vi "Prompt Unflatten Test Parameters.vi"(9 "error in (no error)":errorcluster, 10 "Parameter String":string) -> (1 "error out":errorcluster, 2 "Prompt Test Parameters":T2, 5 "Test Version":string)   [LabVIEW 2011]
uses:
  TypeDefs/Prompt Test Parameters.ctl
  Test Return Parameter.ctl
  TypeDefs/Prompt Test Parameters v1.0-1.4.ctl
  TypeDefs/Prompt Test Parameters v1.5-1.6.ctl
  TypeDefs/Prompt Test Parameters v1.7.ctl
  TypeDefs/Prompt Test Parameters v1.8.ctl
panel:
  in  "Return Parameter":T1
  out "Parameter Variant":variant
  in  "Required Instruments":string[](array[string])
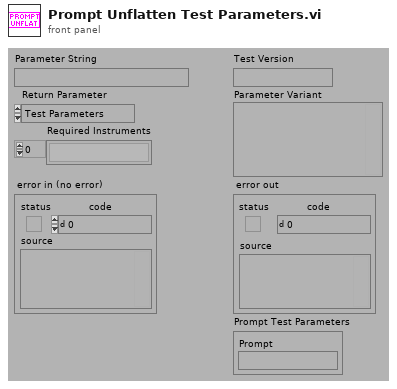
[diagram p1: front panel]
types:
  T1 = typedef "Test Return Parameter.ctl" = enum16{"Test Parameters", "Required Instruments", "Datasheets", "QuickMode"}
  T2 = typedef "Prompt Test Parameters.ctl" = cluster{"Prompt":string}
  T3 = typedef "Prompt Test Parameters v1.0-1.4.ctl" = cluster{"Prompt":string, "Tag":string}
  T4 = typedef "Prompt Test Parameters v1.5-1.6.ctl" = cluster{"Tag":string, "Prompt":string, "Reports":cluster{"Reports to Generate":i32[], "Print Reports":bool}}
  T5 = typedef "Prompt Test Parameters v1.7.ctl" = cluster{"Tag":string, "Prompt":string, "Datasheets":cluster{"Datasheets to Generate":i32[], "Print Datasheets":bool}}
  T6 = typedef "Prompt Test Parameters v1.8.ctl" = cluster{"Prompt":string, "Datasheets":cluster{"Datasheet to Generate":i32, "Print Datasheets":bool}[]}
  T7 = typedef "Test Datasheets v1.0-4.0.ctl" = cluster{"Datasheet to Generate":i32, "Print Datasheets":bool}[]
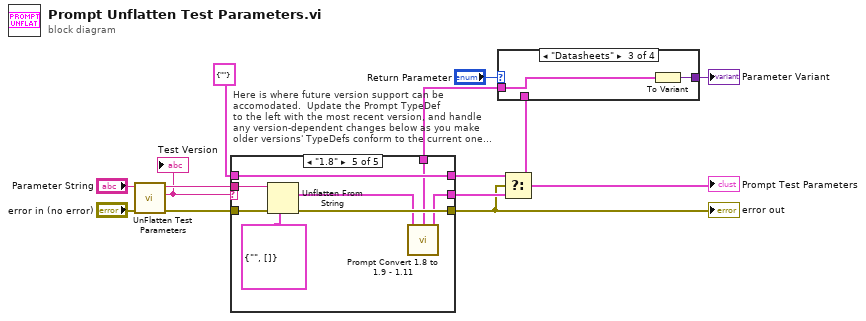
[diagram p0: block diagram]
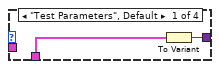
[diagram p2: hidden frame]
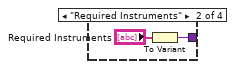
[diagram p3: hidden frame]
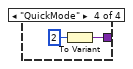
[diagram p4: hidden frame]
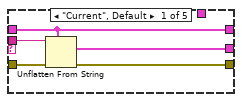
[diagram p5: hidden frame]
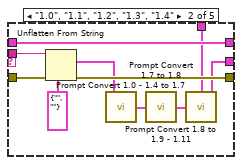
[diagram p6: hidden frame]
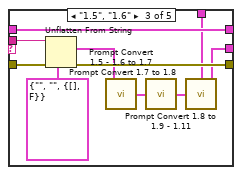
[diagram p7: hidden frame]
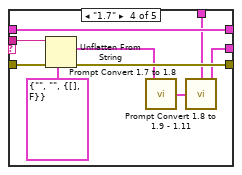
[diagram p8: hidden frame]
diagram:
  # "Here is where future version support can be\naccomodated.  Update the Prompt TypeDef\nto the left with the most recent version, and handle\nany version-dependent changes below as you make\nolder versions' TypeDefs conform to the current one..."
  n1 = call "UnFlatten Test Parameters.vi"("error in (no error)"="error in (no error)", "Flattened Test Parameters with Version (\"\")"="Parameter String") -> ("error out"=w6:errorcluster, "Test Version"=w11:string, "Flat Test Parameters"=w12:string)  [unwired: 3 out]
  "Test Version" <- w11
  n2 = case shown="\"1.8\"" w11 {
    tunnel: [w17 w20 w30 w40 w49] -> w10
    tunnel: T2 {"Prompt"=""} ("Default Prompt Configuration\nMost Current Version") -> [w14 w24 w35 w44 w52]
    tunnel: w12 -> [w18 w28 w38 w47 w55]
    tunnel: [w15 w26 w37 w46 w54] -> w3
    tunnel: w6 -> [w16 w25 w36 w45 w53]
    tunnel: [w14 w24 w35 w44 w52] -> w4
    tunnel: [_ w19 w29 w39 w48] -> w1
    frame "Current", Default {
      n3 = Unflatten From String(type=w14, binary string=w18, error in (no error)=w16) -> (value=w17:T2, error out=w15:errorcluster)  [unwired: 3 out]
    }
    frame "1.0", "1.1", "1.2", "1.3", "1.4" {
      n4 = Unflatten From String(type=T3 {"Prompt"="", "Tag"=""} ("Prompt Parameters"), binary string=w28, error in (no error)=w25) -> (value=w22:T3, error out=w26:errorcluster)  [unwired: 3 out]
      n5 = call "Prompt Convert 1.0 - 1.4 to 1.7.vi"("Prompt 1.0 - 1.4 Test Parameters"=w22) -> ("Prompt 1.7 Test Parameters"=w23:T5)
      n6 = call "Prompt Convert 1.7 to 1.8.vi"("Prompt 1.7 Test Parameters"=w23) -> ("Prompt 1.8 Test Parameters"=w21:T6)
      n7 = call "Prompt Convert 1.8 to 1.9 - 1.11.vi"("Prompt 1.8 Test Parameters"=w21) -> ("Datasheets"=w19:T7, "Prompt 1.9 - 1.11 Test Parameters"=w20:T2)
    }
    frame "1.5", "1.6" {
      n8 = Unflatten From String(type=T4 {"Tag"="", "Prompt"="", "Reports"={"Reports to Generate"=[], "Print Reports"=FALSE}} ("Prompt Test Parameters"), binary string=w38, error in (no error)=w36) -> (value=w33:T4, error out=w37:errorcluster)  [unwired: 3 out]
      n9 = call "Prompt Convert 1.5 - 1.6 to 1.7.vi"("Prompt 1.5 - 1.6 Test Parameters"=w33) -> ("Prompt 1.7 Test Parameters"=w32:T5)
      n10 = call "Prompt Convert 1.7 to 1.8.vi"("Prompt 1.7 Test Parameters"=w32) -> ("Prompt 1.8 Test Parameters"=w31:T6)
      n11 = call "Prompt Convert 1.8 to 1.9 - 1.11.vi"("Prompt 1.8 Test Parameters"=w31) -> ("Datasheets"=w29:T7, "Prompt 1.9 - 1.11 Test Parameters"=w30:T2)
    }
    frame "1.7" {
      n12 = Unflatten From String(type=T5 {"Tag"="", "Prompt"="", "Datasheets"={"Datasheets to Generate"=[], "Print Datasheets"=FALSE}} ("Prompt Test Parameters"), binary string=w47, error in (no error)=w45) -> (value=w42:T5, error out=w46:errorcluster)  [unwired: 3 out]
      n13 = call "Prompt Convert 1.7 to 1.8.vi"("Prompt 1.7 Test Parameters"=w42) -> ("Prompt 1.8 Test Parameters"=w41:T6)
      n14 = call "Prompt Convert 1.8 to 1.9 - 1.11.vi"("Prompt 1.8 Test Parameters"=w41) -> ("Datasheets"=w39:T7, "Prompt 1.9 - 1.11 Test Parameters"=w40:T2)
    }
    frame "1.8" {
      n15 = Unflatten From String(type=T6 {"Prompt"="", "Datasheets"=[]} ("Prompt Test Parameters"), binary string=w55, error in (no error)=w53) -> (value=w50:T6, error out=w54:errorcluster)  [unwired: 3 out]
      n16 = call "Prompt Convert 1.8 to 1.9 - 1.11.vi"("Prompt 1.8 Test Parameters"=w50) -> ("Datasheets"=w48:T7, "Prompt 1.9 - 1.11 Test Parameters"=w49:T2)
    }
  }
  "error out" <- w3
  n17 = Select(t=w4, s=w3, f=w10) -> (s? t:f=w2:T2)
  "Prompt Test Parameters" <- w2
  n18 = case shown="\"Datasheets\"" "Return Parameter" {
    tunnel: [w57 w59 w61 w63] -> w8
    tunnel: w2 -> [w56 _ _ _]
    tunnel: w1 -> [_ _ w60 _]
    frame "Test Parameters", Default {
      n19 = To Variant(anything=w56) -> (Variant=w57:variant)
    }
    frame "Required Instruments" {
      n20 = To Variant(anything="Required Instruments") -> (Variant=w59:variant)
    }
    frame "Datasheets" {
      n21 = To Variant(anything=w60) -> (Variant=w61:variant)
    }
    frame "QuickMode" {
      n22 = To Variant(anything=i8 2 ("QuickMode")) -> (Variant=w63:variant)
    }
  }
  "Parameter Variant" <- w8
